vi "Create User Events - ExitMultiLoop.vi"(8 "error in (no error)":errorcluster) -> (0 "error out":errorcluster, 1 "ExitALLLoops event out":refnum<user-event>, 2 "ExitEventLoop event out":refnum<user-event>, 3 "Events Registration Refnum":refnum<event-registration>, 5 "user event array":refnum<user-event>[](array[refnum]))   [LabVIEW 2018, in "UserEvent-ExitEventLoop.lvlib"]
doc: "Create a boolean user event that will be used to stop the event loop from the message handling loop.\nCreate a boolean user event that will be used to stop ALL loops in a muliploop statemachines VI.\n\nBolder Software LLC"
uses:
  UserEvent-ExitEventLoop.lvlib
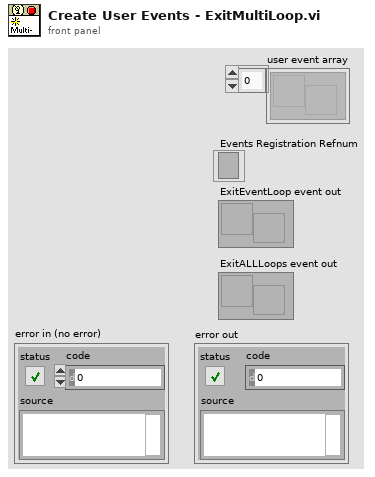
[diagram p1: front panel]
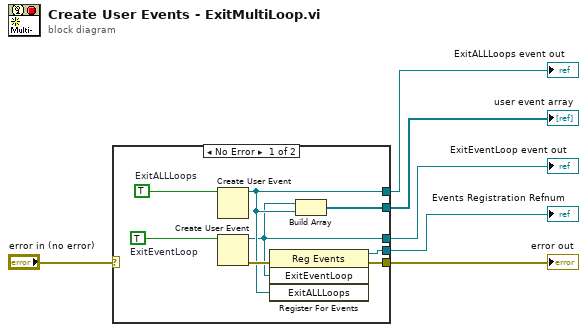
[diagram p0: block diagram]
diagram:
  n1 = case shown="No Error" "error in (no error)" {
    selector: "error in (no error)" -> [_ w15]
    tunnel: [w10 _] -> w6
    tunnel: [w12 w15] -> w5
    tunnel: [w9 _] -> w3
    tunnel: [w8 _] -> w2
    tunnel: [w7 _] -> w1
    frame No Error {
      w11 = TRUE  # ExitALLLoops
      w13 = TRUE  # ExitEventLoop
      n2 = Create User Event(user event datatype=w11) -> (user event=w8:refnum<user-event>)  [unwired: 1 in, 1 out]
      n3 = Create User Event(user event datatype=w13) -> (user event=w7:refnum<user-event>, error out=w14:errorcluster)  [unwired: 1 in]
      n4 = register-events(error in=w14, w7, w8) -> (reference out=w10:refnum<event-registration>, error out=w12:errorcluster)  [unwired: 1 in]
      n5 = Build Array(w7, w8) -> (w9:refnum<user-event>[])
    }
    frame Error {
    }
  }
  "Events Registration Refnum" <- w6
  "user event array" <- w3
  "error out" <- w5
  "ExitEventLoop event out" <- w1
  "ExitALLLoops event out" <- w2
